vi "RegularExpressionEscape.vi"(11 "String":string) -> (3 "result string":string)   [LabVIEW 2019]
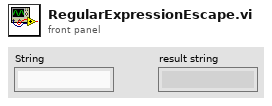
[diagram p1: front panel]
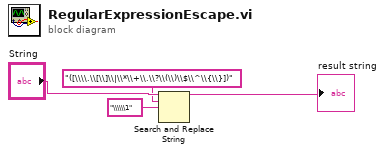
[diagram p0: block diagram]
diagram:
  n1 = Search and Replace String(input string="String", search string="([\\\\.\\[\\]\\|\\*\\+\\.\\?\\(\\)\\$\\^\\{\\}])", replace string="\\\\\\1" ("replace string (\"\")")) -> (result string=→"result string":string)  [unwired: 5 in, 3 out]
